vi "Finish.vi"   [LabVIEW 2016]
doc: "This VI is called just before exiting. It is expected to close I/O refnum, save collected data, etc."
uses:
  <vilib>/Rock Robotics/WPI/Utilities/WPI_GetSetVariantRefNum.vi
types:
  T1 = typedef "WPI_JoystickDevRef.ctl" = cluster{"Device":T2}
  T2 = typedef "WPI_JoystickDeviceEnum.ctl" = enum16{"USB 0", "USB 1", "USB 2", "USB 3", "USB 4", "USB 5"}
  T3 = typedef "WPI_MotorControlDeviceRef.ctl" = cluster{"DeviceStatus":errorcluster, "Type":T4, "PWM":cluster{"PWM Channel":T5, "DeadBand":T6}, "CAN":cluster{"Device Number":u8, "SetOutput VI Ref":variant, "GetOutput VI Ref":variant, "Enable VI Ref":variant, "Disable VI Ref":variant, "Data":variant}, "Invert":bool}
  T4 = typedef "WPI_MotorControlType.ctl" = enum16{"PWM", "CAN"}
  T5 = typedef "FPGA_DIOPWMChannel.ctl" = enum8{"PWM 0", "PWM 1", "PWM 2", "PWM 3", "PWM 4", "PWM 5", "PWM 6", "PWM 7", "PWM 8", "PWM 9", "PWM MXP 0", "PWM MXP 1", "PWM MXP 2", "PWM MXP 3", "PWM MXP 4", "PWM MXP 5", "PWM MXP 6", "PWM MXP 7", "PWM MXP 8", "PWM MXP 9", "Invalid"}
  T6 = typedef "WPI_PWMDeadband.ctl" = cluster{"Name":string, "maxPositivePwm":i32, "minPositivePwm":i32, "centerPwm":i32, "maxNegativePwm":i32, "minNegativePwm":i32, "angularRange":u16}
  T7 = typedef "WPI_CompressorDevRef.ctl" = cluster{"DevStatus":errorcluster, "Pneumatics Control Module":u8}
  T8 = typedef "WPI_SolenoidDevRef.ctl" = cluster{"DevStatus":errorcluster, "Pneumatics Control Module":u8, "Forward Solenoid Channel":T9, "Reverse Solenoid Channel":T9}
  T9 = typedef "WPI_SolenoidChannel.ctl" = enum8{"Solenoid 0", "Solenoid 1", "Solenoid 2", "Solenoid 3", "Solenoid 4", "Solenoid 5", "Solenoid 6", "Solenoid 7", "Invalid"}
  T10 = typedef "WPI_RobotDriveDevRef.ctl" = cluster{"DevStatus":errorcluster, "Motors[]":T3[], "Square Inputs":bool, "Max Output":dbl}
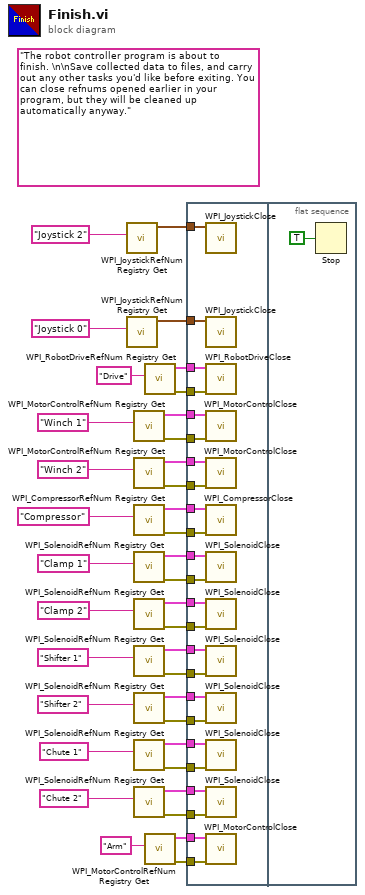
[diagram p0: block diagram]
diagram:
  (unwired) "The robot controller program is about to finish. \n\nSave collected data to files, and carry out any other tasks you'd like before exiting. You can close refnums opened earlier in your program, but they will be cleaned up automatically anyway."
  n1 = call <vilib>:"WPI_JoystickRefNum Registry Get.vi"("refnum name"="Joystick 2") -> ("JoystickDevRef"=w34:T1)  [unwired: 1 in, 9 out]
  n2 = call <vilib>:"WPI_JoystickRefNum Registry Get.vi"("refnum name"="Joystick 0") -> ("JoystickDevRef"=w36:T1)  [unwired: 1 in, 9 out]
  n3 = call <vilib>:"WPI_MotorControlRefNum Registry Get.vi"("refnum name"="Winch 1") -> ("error out"=w28:errorcluster, "MotorControlDevRef"=w27:T3)  [unwired: 9 in]
  n4 = call <vilib>:"WPI_MotorControlRefNum Registry Get.vi"("refnum name"="Winch 2") -> ("error out"=w25:errorcluster, "MotorControlDevRef"=w26:T3)  [unwired: 9 in]
  n5 = call <vilib>:"WPI_CompressorRefNum Registry Get.vi"("refnum name"="Compressor") -> ("error out"=w23:errorcluster, "CompressorDevRef"=w24:T7)  [unwired: 9 in]
  n6 = call <vilib>:"WPI_SolenoidRefNum Registry Get.vi"("refnum name"="Clamp 1") -> ("error out"=w17:errorcluster, "SolenoidDevRef"=w18:T8)  [unwired: 9 in]
  n7 = call <vilib>:"WPI_SolenoidRefNum Registry Get.vi"("refnum name"="Clamp 2") -> ("error out"=w9:errorcluster, "SolenoidDevRef"=w10:T8)  [unwired: 9 in]
  n8 = call <vilib>:"WPI_SolenoidRefNum Registry Get.vi"("refnum name"="Shifter 1") -> ("error out"=w7:errorcluster, "SolenoidDevRef"=w8:T8)  [unwired: 9 in]
  n9 = call <vilib>:"WPI_SolenoidRefNum Registry Get.vi"("refnum name"="Shifter 2") -> ("error out"=w5:errorcluster, "SolenoidDevRef"=w6:T8)  [unwired: 9 in]
  n10 = call <vilib>:"WPI_SolenoidRefNum Registry Get.vi"("refnum name"="Chute 1") -> ("error out"=w3:errorcluster, "SolenoidDevRef"=w4:T8)  [unwired: 9 in]
  n11 = call <vilib>:"WPI_SolenoidRefNum Registry Get.vi"("refnum name"="Chute 2") -> ("error out"=w1:errorcluster, "SolenoidDevRef"=w2:T8)  [unwired: 9 in]
  n12 = call <vilib>:"WPI_RobotDriveRefNum Registry Get.vi"("refnum name"="Drive") -> ("error out"=w20:errorcluster, "RobotDriveDevRef"=w21:T10)  [unwired: 9 in]
  n13 = call <vilib>:"WPI_MotorControlRefNum Registry Get.vi"("refnum name"="Arm") -> ("error out"=w29:errorcluster, "MotorControlDevRef"=w30:T3)  [unwired: 9 in]
  n14 = flat-sequence {
    tunnel: w36 -> [w61]
    tunnel: w34 -> [w60]
    tunnel: w30 -> [w59]
    tunnel: w29 -> [w58]
    tunnel: w28 -> [w57]
    tunnel: w27 -> [w56]
    tunnel: w26 -> [w55]
    tunnel: w25 -> [w54]
    tunnel: w24 -> [w53]
    tunnel: w23 -> [w52]
    tunnel: w21 -> [w51]
    tunnel: w20 -> [w50]
    tunnel: w18 -> [w49]
    tunnel: w17 -> [w48]
    tunnel: w10 -> [w47]
    tunnel: w9 -> [w46]
    tunnel: w8 -> [w45]
    tunnel: w7 -> [w44]
    tunnel: w6 -> [w43]
    tunnel: w5 -> [w42]
    tunnel: w4 -> [w41]
    tunnel: w3 -> [w40]
    tunnel: w2 -> [w39]
    tunnel: w1 -> [w38]
    frame #0 {
      n15 = call <vilib>:"WPI_JoystickClose.vi"("JoystickDevRef"=w60) -> ()  [unwired: 11 out]
      n16 = call <vilib>:"WPI_JoystickClose.vi"("JoystickDevRef"=w61) -> ()  [unwired: 11 out]
      n17 = call <vilib>:"WPI_RobotDriveClose.vi"("error in (no error)"=w50, "RobotDriveDevRef"=w51) -> ()  [unwired: 9 in, 1 out]
      n18 = call <vilib>:"WPI_MotorControlClose.vi"("error in"=w57, "MotorControlDevRef"=w56) -> ()  [unwired: 9 in, 1 out]
      n19 = call <vilib>:"WPI_MotorControlClose.vi"("error in"=w54, "MotorControlDevRef"=w55) -> ()  [unwired: 9 in, 1 out]
      n20 = call <vilib>:"WPI_CompressorClose.vi"("error in (no error)"=w52, "CompressorDevRef"=w53) -> ()  [unwired: 9 in, 1 out]
      n21 = call <vilib>:"WPI_SolenoidClose.vi"("error in (no error)"=w48, "SolenoidDevRef"=w49) -> ()  [unwired: 9 in, 1 out]
      n22 = call <vilib>:"WPI_SolenoidClose.vi"("error in (no error)"=w46, "SolenoidDevRef"=w47) -> ()  [unwired: 9 in, 1 out]
      n23 = call <vilib>:"WPI_SolenoidClose.vi"("error in (no error)"=w44, "SolenoidDevRef"=w45) -> ()  [unwired: 9 in, 1 out]
      n24 = call <vilib>:"WPI_SolenoidClose.vi"("error in (no error)"=w42, "SolenoidDevRef"=w43) -> ()  [unwired: 9 in, 1 out]
      n25 = call <vilib>:"WPI_SolenoidClose.vi"("error in (no error)"=w40, "SolenoidDevRef"=w41) -> ()  [unwired: 9 in, 1 out]
      n26 = call <vilib>:"WPI_SolenoidClose.vi"("error in (no error)"=w38, "SolenoidDevRef"=w39) -> ()  [unwired: 9 in, 1 out]
      n27 = call <vilib>:"WPI_MotorControlClose.vi"("error in"=w58, "MotorControlDevRef"=w59) -> ()  [unwired: 9 in, 1 out]
    }
    frame #1 {
      n28 = Stop(stop? (T)=TRUE ("Quit")) -> ()
    }
  }
